vi "Code that needs to be put in autonomous.vi"() -> ()   [LabVIEW 2015]
uses:
  <vilib>/Rock Robotics/Network Tables/NT Read Number.vi
  Framework/Robot Global Data.vi
  navX Library v2/navX Library v2.lvlib
panel:
  in  "Pitch tolerance while driving on flat ground":dbl=5.0 format="%#_13g"
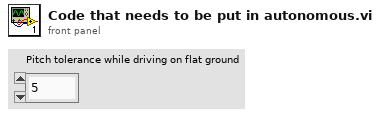
[diagram p1: front panel]
types:
  T1 = typedef "navX Library v2.lvlib/Z900_navX_DeviceTypeDef.ctl" = cluster{"Interface":cluster{"Protocol":T2, "Update Rate (4Hz-60Hz)":u8, "navX Open TypeDef":variant}, "Notify Packet":refnum<notifier>, "Loop VI Refnum":refnum<vi>, "Ready to Close Occurrence Refnum":refnum<k4>}
  T2 = typedef "navX Library v2.lvlib/Z900_navX_ProtocolTypeDef.ctl" = enum16{"SERIAL", "I2C", "SPI"}
  T3 = cluster{"Yaw":dbl, "Roll":dbl, "Pitch":dbl, "Heading":dbl, "Fused Heading":dbl}
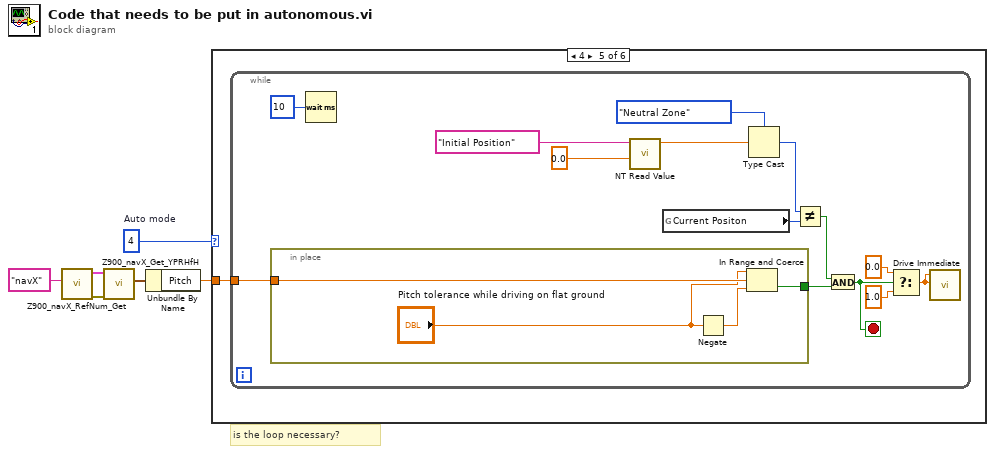
[diagram p0: block diagram]
diagram:
  w6 = 4  # Auto mode
  # "is the loop necessary?"
  n1 = call "Z900_navX_RefNum_Get.vi"("refnum name"="navX") -> ("error out"=w3:errorcluster, "navX Device"=w4:T1)  [unwired: 9 in]
  n2 = call "Z900_navX_Get_YPRHfH.vi"("error in (no error)"=w3, "navX Device"=w4) -> ("YRPHfH"=w2:T3)  [unwired: 6 in, 3 out]
  n3 = Unbundle By Name(w2) -> ("Pitch"=w1:dbl)
  n4 = case shown="4" w6 {
    tunnel: w1 -> [_ _ _ _ w7 _]
    frame 0, Default {
    }
    frame 1 {
    }
    frame 2 {
    }
    frame 3 {
    }
    frame 4 {
      n5 = while {
        tunnel: w7 -> [w10]
        stop <- w9 stop-if-true
        n6 = in-place {
          in-place-border: w10 -> [w25]
          in-place-border: [w22] -> w14
          n7 = Negate(x="Pitch tolerance while driving on flat ground") -> (-x=w23:dbl)
          n8 = In Range and Coerce(upper limit="Pitch tolerance while driving on flat ground", x=w25, lower limit=w23) -> (In Range?=w22:bool)  [unwired: 1 out]
        }
        n9 = Wait (ms)(milliseconds to wait=u32 10) -> ()  [unwired: 1 out]
        n10 = call-poly <vilib>:"NT Read Value.vi"("Default Value"=0.0, "Name"="Initial Position") -> ("Numeric"=w18:dbl)  [unwired: 8 in, 1 out]
        n11 = global read "Robot Global Data.vi" "Current Positon"() -> (w16:enum16{"Neutral Zone", "Courtyard"})
        n12 = Type Cast(type=enum16{"Neutral Zone", "Courtyard"}."Neutral Zone" ("Current Positon 2"), x=w18) -> (*(type *) &x=w17:enum16{"Neutral Zone", "Courtyard"})
        n13 = Not Equal?(x=w17, y=w16) -> (x != y?=w15:bool)
        n14 = And(x=w15, y=w14) -> (x .and. y?=w9:bool)
        n15 = Select(t=0.0, s=w9, f=1.0) -> (s? t:f=w12:dbl)
        n16 = call "Drive Immediate.vi"("Right Setpoint"=w12, "Left Setpoint"=w12) -> ()  [unwired: 9 in, 1 out]
      }
    }
    frame 5 {
    }
  }
